vi "MALT WriteRead.vi"(8 "error in":errorcluster, 11 "Request":string="SAY_HELLO_WOLRD") -> (0 "error out":errorcluster, 3 "Response":string)   [LabVIEW 2018]
uses:
  Global/MALT Global.vi
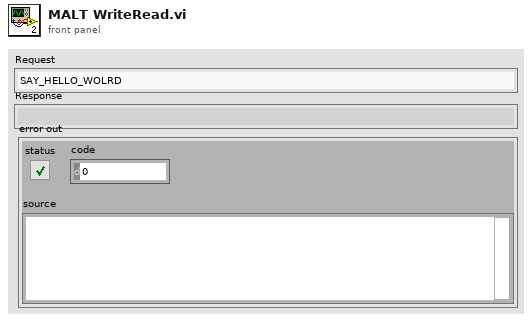
[diagram p1: front panel]
types:
  T1 = enum16{"Standard", "Buffered", "CRLF", "Immediate"}
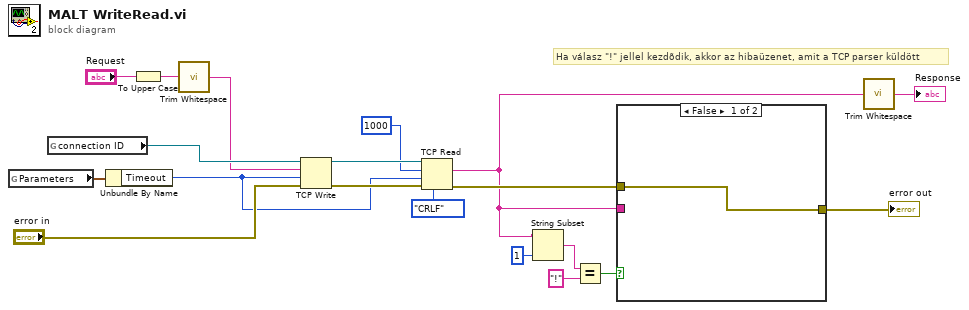
[diagram p0: block diagram]
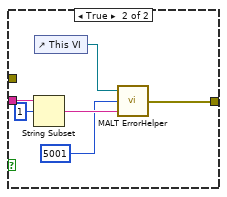
[diagram p2: hidden frame]
diagram:
  # "Ha válasz \"!\" jellel kezdõdik, akkor az hibaüzenet, amit a TCP parser küldött"
  n1 = global read "MALT Global.vi" "Parameters"() -> (w13:cluster{"Timeout":i32})
  n2 = global read "MALT Global.vi" "connection ID"() -> (w14:refnum<k5>)
  n3 = Unbundle By Name(w13) -> ("Timeout"=w8:i32)
  n4 = To Upper Case(1:"Request") -> (0:w12:string)
  n5 = call <vilib>:"Trim Whitespace.vi"("string"=w12) -> ("trimmed string"=w10:string)  [unwired: 1 in]
  n6 = TCP Write(connection ID=w14, data in=w10, error in (no error)="error in", 9:w8) -> (connection ID out=w19:refnum<k5>, error out=w16:errorcluster)  [unwired: 1 out]
  n7 = TCP Read(connection ID=w19, bytes to read=1000, error in (no error)=w16, 7:T1."CRLF" ("mode (standard)"), 9:w8) -> (data out=w2:string, error out=w3:errorcluster)  [unwired: 1 out]
  n8 = String Subset(string=w2, length (rest)=1 ("length (rest)")) -> (substring=w6:string)  [unwired: 1 in]
  n9 = Equal?(x=w6, y="!") -> (x = y?=w4:bool)
  n10 = case shown="False" w4 {
    tunnel: w3 -> [w20 _]
    tunnel: w2 -> [_ w25]
    tunnel: [w20 w21] -> w1
    frame False {
    }
    frame True {
      n11 = String Subset(string=w25, offset (0)=1) -> (substring=w23:string)  [unwired: 1 in]
      n12 = control-ref of="This VI"() -> (w26:refnum<vi>)
      n13 = call "MALT ErrorHelper.vi"("Message"=w23, "Code"=5001, "This VI"=w26) -> ("error out"=w21:errorcluster)
    }
  }
  "error out" <- w1
  n14 = call <vilib>:"Trim Whitespace.vi"("string"=w2) -> ("trimmed string"=→"Response":string)  [unwired: 1 in]
